vi "example_GMotionComplete.vi"() -> ()   [LabVIEW 2021]
uses:
  <vilib>/Galil/resources/gclib/gclib.lvlib
  <vilib>/Galil/resources/gclibo/gclibo.lvlib
panel:
  out "Reference Position":string
  in  "Command 2":string="MG_RPA"
  out "Error Out":errorcluster
  in  "IP Address":string="192.168.1.77"
  in  "Command":string="SHA;PRA=4000;BGA"
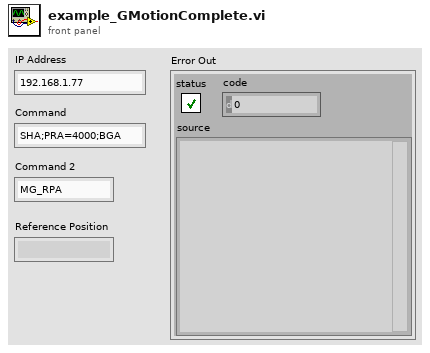
[diagram p1: front panel]
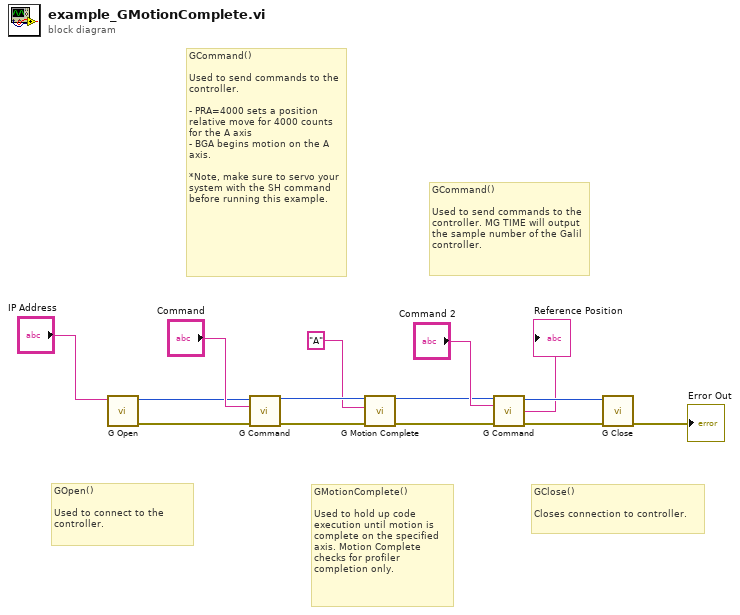
[diagram p0: block diagram]
diagram:
  # "GCommand()\n\nUsed to send commands to the controller. MG TIME will output the sample number of the Galil controller."
  # "GMotionComplete()\n\nUsed to hold up code execution until motion is complete on the specified axis. Motion Complete checks for profiler completion only."
  # "GClose()\n\nCloses connection to controller."
  # "GCommand()\n\nUsed to send commands to the controller. \n\n- PRA=4000 sets a position relative move for 4000 counts for the A axis\n- BGA begins motion on the A axis.\n\n*Note, make sure to servo your system with the SH command before running this example."
  # "GOpen()\n\nUsed to connect to the controller."
  n1 = call <vilib>:"G Open.vi"("address"="IP Address") -> ("error out"=w1:errorcluster, "g out"=w3:u64)  [unwired: 8 in]
  n2 = call <vilib>:"G Command.vi"("g"=w3, "command"="Command", "error in (no error)"=w1) -> ("g out"=w9:u64, "error out"=w7:errorcluster)  [unwired: 10 in, 1 out]
  n3 = call <vilib>:"G Motion Complete.vi"("error in (no error)"=w7, "axes"="A", "g"=w9) -> ("error out"=w6:errorcluster, "g out"=w8:u64)  [unwired: 7 in]
  n4 = call <vilib>:"G Command.vi"("g"=w8, "command"="Command 2", "error in (no error)"=w6) -> ("g out"=w12:u64, "buffer out"=→"Reference Position":string, "error out"=w11:errorcluster)  [unwired: 10 in]
  n5 = call <vilib>:"G Close.vi"("error in (no error)"=w11, "g"=w12) -> ("error out"=→"Error Out":errorcluster)  [unwired: 9 in]
